vi "Read Sinus penta1.vi"(10 "Parametri inverter 2":T1, 11 "register values":u16[](array[numeric])) -> (2 "output cluster":T1)   [LabVIEW 2019]
uses:
  controls/Parametri inverter letti.ctl
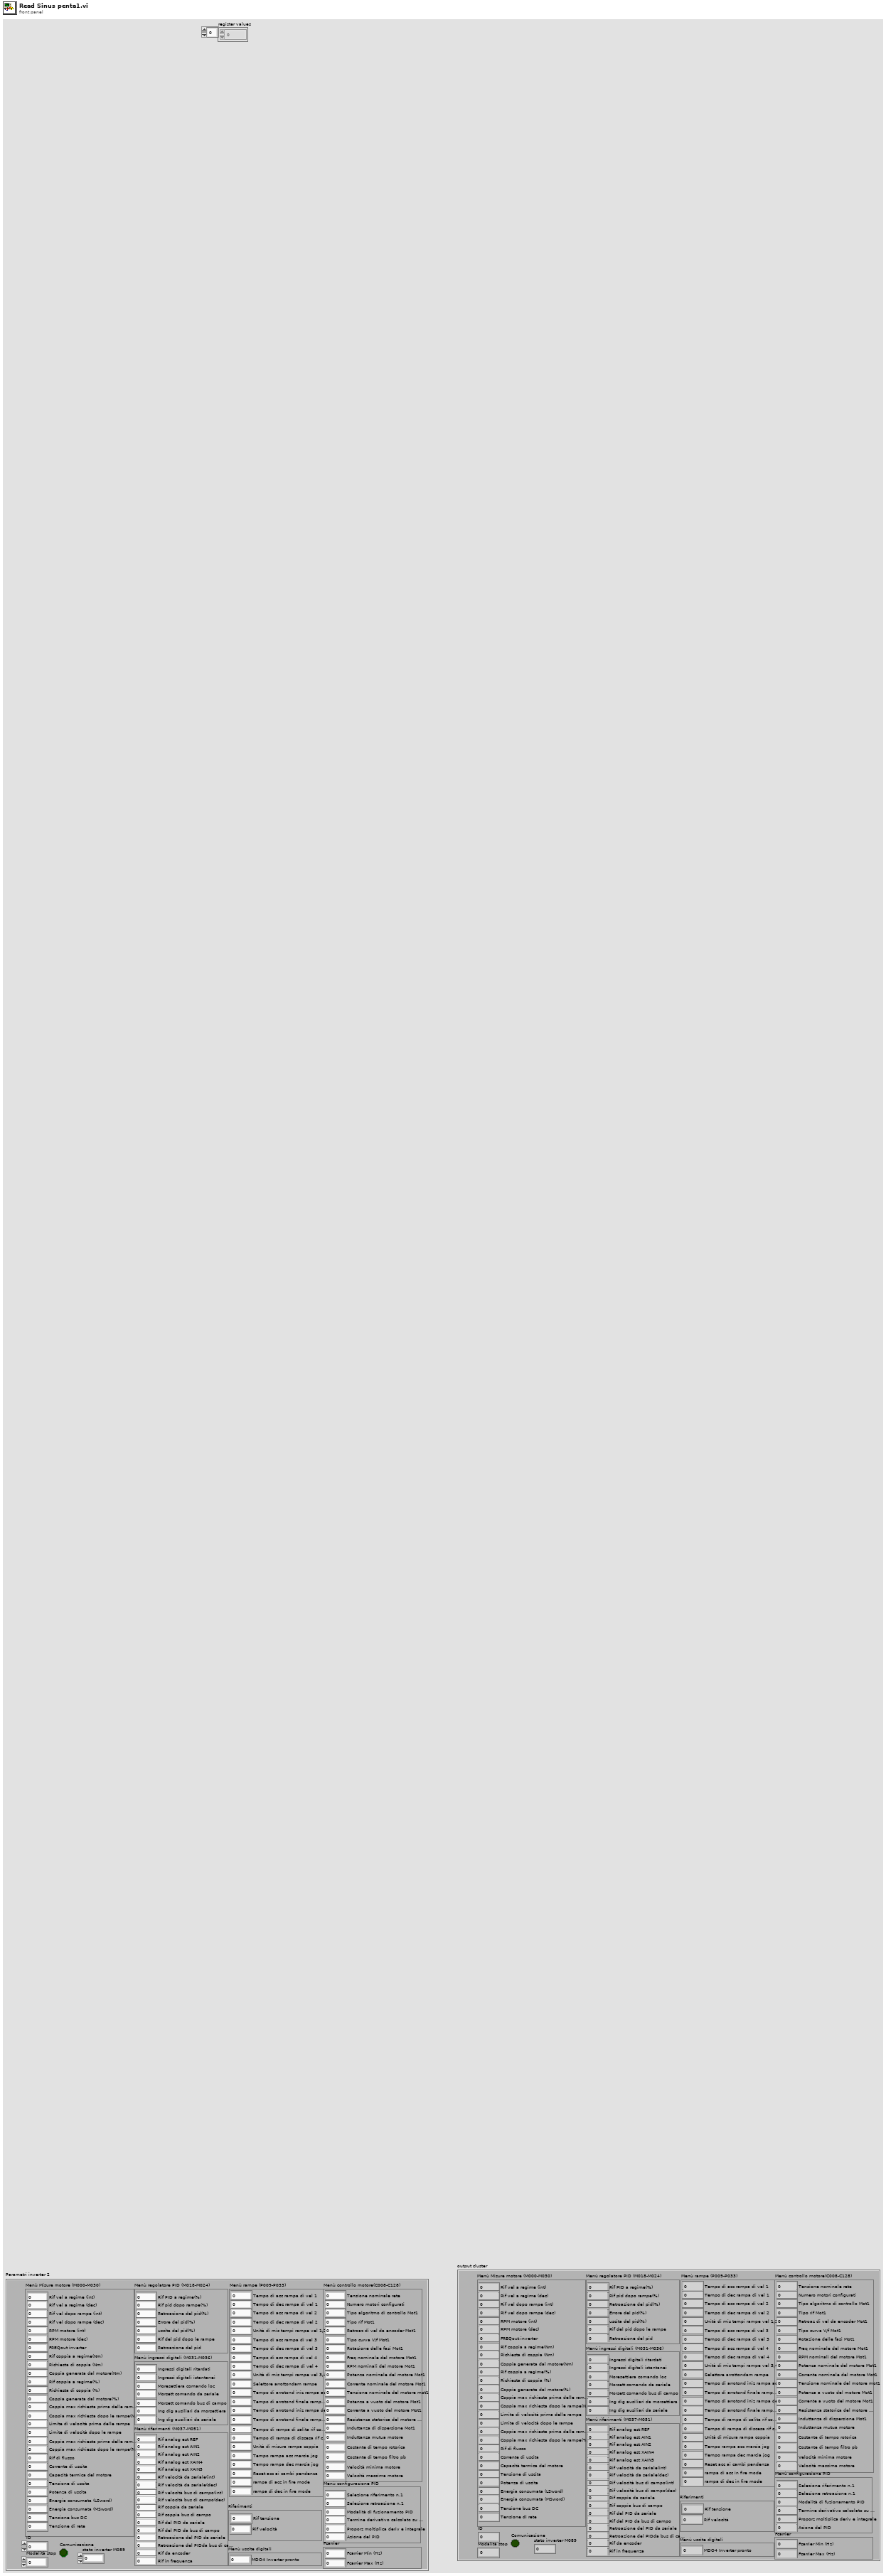
[diagram p1: front panel]
types:
  T1 = typedef "Parametri inverter letti.ctl" = cluster{"Menù Misure motore (M000-M030)":cluster{"Rif vel a regime (int)":u16, "Rif vel a regime (dec)":u16, "Rif vel dopo rampe (int)":u16, "Rif vel dopo rampe (dec)":u16, "RPM motore (int)":u16, "RPM motore (dec)":u16, "FREQout inverter":u16, "Rif coppia a regime(Nm)":u16, "Richiesta di coppia (Nm)":u16, "Coppia generata dal motore(Nm)":u16, "Rif coppia a regime(%)":u16, "Richiesta di coppia (%)":u16, "Coppia generata dal motore(%)":u16, "Coppia max richiesta prima delle rampe(Nm)":u16, "Coppia max richiesta dopo le rampe(Nm)":u16, "Limite di velocità prima delle rampe":u16, "Limite di velocità dopo le rampe":u16, "Coppia max richiesta prima delle rampe(%)":u16, "Coppia max richiesta dopo le rampe(%)":u16, "Rif di flusso":u16, "Corrente di uscita":u16, "Capacità termica del motore":u16, "Tensione di uscita":u16, "Potenza di uscita":u16, "Energia consumata (LSword)":u16, "Energia consumata (MSword)":u16, "Tensione bus DC":u16, "Tensione di rete":u16}, "Menù regolatore PID (M018-M024)":cluster{"Rif PID a regime(%)":u16, "Rif pid dopo rampe(%)":u16, "Retroazione del pid(%)":u16, "Errore del pid(%)":u16, "uscita del pid(%)":u16, "Rif del pid dopo le rampe":u16, "Retroazione del pid":u16}, "Menù ingressi digitali (M031-M036)":cluster{"Ingressi digitali ritardati":u16, "Ingressi digitali istantanei":u16, "Moresettiera comando loc":u16, "Morsett comando da seriale":u16, "Morsett comando bus di campo":u16, "Ing dig ausiliari da morsettiera":u16, "Ing dig ausiliari da seriale":u16}, "Menù riferimenti (M037-M051)":cluster{"Rif analog est REF":u16, "Rif analog est AIN1":u16, "Rif analog est AIN2":u16, "Rif analog est XAIN4":u16, "Rif analog est XAIN5":u16, "Rif velocità da seriale(int)":u16, "Rif velocità bus di campo(int)":u16, "Rif coppia da seriale":u16, "Rif coppia bus di campo":u16, "Rif del PID da seriale":u16, "Rif del PID da bus di campo":u16, "Retroazione del PID da seriale":u16, "Retroazione del PIDda bus di campo":u16, "Rif da encoder":u16, "Rif in frequenza":u16, "Rif velocità da seriale(dec)":u16, "Rif velocità bus di campo(dec)":u16}, "Menù rampe (P009-P033)":cluster{"Tempo di dec rampa di vel 1":u16, "Tempo di acc rampa di vel 2":u16, "Tempo di dec rampa di vel 2":u16, "Tempo di acc rampa di vel 1":u16, "Unità di mis tempi rampe vel 1/2":u16, "Tempo di acc rampa di vel 3":u16, "Tempo di dec rampa di vel 3":u16, "Tempo di acc rampa di vel 4":u16, "Tempo di dec rampa di vel 4":u16, "Unità di mis tempi rampe vel 3/4":u16, "Selettore arrottondam rampe":u16, "Tempo di arrotond iniz rampa acc":u16, "Tempo di arrotond finale rampa acc":u16, "Tempo di arrotond iniz rampa dec":u16, "Tempo di rampa di salita rif coppia":u16, "Tempo di rampa di discesa rif coppia":u16, "Unità di misura rampa coppia":u16, "Tempo rampa acc marcia jog":u16, "Tempo rampa dec marcia jog":u16, "Reset acc ai cambi pendenza":u16, "rampa di acc in fire mode":u16, "rampa di dec in fire mode":u16, "Tempo di arrotond finale rampa dec":u16}, "Menù controllo motore(C008-C128)":cluster{"Numero motori configurati":u16, "Tipo algoritmo di controllo Mot1":u16, "Tipo rif Mot1":u16, "Tensione nominale rete":u16, "Retroaz di vel da encoder Mot1":u16, "Tipo curva V/f Mot1":u16, "Rotazione delle fasi Mot1":u16, "Freq nominale del motore Mot1":u16, "RPM nominali del motore Mot1":u16, "Potenza nominale del motore Mot1":u16, "Corrente nominale del motore Mot1":u16, "Tensione nominale del motore mot1":u16, "Potenza a vuoto del motore Mot1":u16, "Corrente a vuoto del motore Mot1":u16, "Resistenza statorica del motore Mot1":u16, "Induttanza di dispersione Mot1":u16, "Induttanza mutua motore":u16, "Costante di tempo rotorica":u16, "Costante di tempo filtro pb":u16, "Velocità minima motore":u16, "Velocità massima motore":u16}, "Menù configurazione PID":cluster{"Selezione riferimento n.1":u16, "Selezione retroazione n.1":u16, "Modalità di fuzionamento PID":u16, "Termine derivativo calcolato su err o mis":u16, "Proporz moltiplica deriv e integrale":u16, "Azione del PID":u16}, "ID":dbl, "Menù uscite digitali":cluster{"MDO4 Inverter pronto":u16}, "Fcarrier":cluster{"Fcarrier Min (Hz)":u16, "Fcarrier Max (Hz)":u16}, "stato inverter M089":dbl, "Riferimenti":cluster{"Rif tensione":u16, "Rif velocità":u16}, "Comunicazione":bool, "Modalità stop":dbl}
  T2 = cluster{"Rif PID a regime(%)":u16, "Rif pid dopo rampe(%)":u16, "Retroazione del pid(%)":u16, "Errore del pid(%)":u16, "uscita del pid(%)":u16, "Rif del pid dopo le rampe":u16, "Retroazione del pid":u16}
  T3 = cluster{"Ingressi digitali ritardati":u16, "Ingressi digitali istantanei":u16, "Moresettiera comando loc":u16, "Morsett comando da seriale":u16, "Morsett comando bus di campo":u16, "Ing dig ausiliari da morsettiera":u16, "Ing dig ausiliari da seriale":u16}
  T4 = cluster{"Rif vel a regime (int)":u16, "Rif vel a regime (dec)":u16, "Rif vel dopo rampe (int)":u16, "Rif vel dopo rampe (dec)":u16, "RPM motore (int)":u16, "RPM motore (dec)":u16, "FREQout inverter":u16, "Rif coppia a regime(Nm)":u16, "Richiesta di coppia (Nm)":u16, "Coppia generata dal motore(Nm)":u16, "Rif coppia a regime(%)":u16, "Richiesta di coppia (%)":u16, "Coppia generata dal motore(%)":u16, "Coppia max richiesta prima delle rampe(Nm)":u16, "Coppia max richiesta dopo le rampe(Nm)":u16, "Limite di velocità prima delle rampe":u16, "Limite di velocità dopo le rampe":u16, "Coppia max richiesta prima delle rampe(%)":u16, "Coppia max richiesta dopo le rampe(%)":u16, "Rif di flusso":u16, "Corrente di uscita":u16, "Capacità termica del motore":u16, "Tensione di uscita":u16, "Potenza di uscita":u16, "Energia consumata (LSword)":u16, "Energia consumata (MSword)":u16, "Tensione bus DC":u16, "Tensione di rete":u16}
  T5 = cluster{"Rif analog est REF":u16, "Rif analog est AIN1":u16, "Rif analog est AIN2":u16, "Rif analog est XAIN4":u16, "Rif analog est XAIN5":u16, "Rif velocità da seriale(int)":u16, "Rif velocità bus di campo(int)":u16, "Rif coppia da seriale":u16, "Rif coppia bus di campo":u16, "Rif del PID da seriale":u16, "Rif del PID da bus di campo":u16, "Retroazione del PID da seriale":u16, "Retroazione del PIDda bus di campo":u16, "Rif da encoder":u16, "Rif in frequenza":u16, "Rif velocità da seriale(dec)":u16, "Rif velocità bus di campo(dec)":u16}
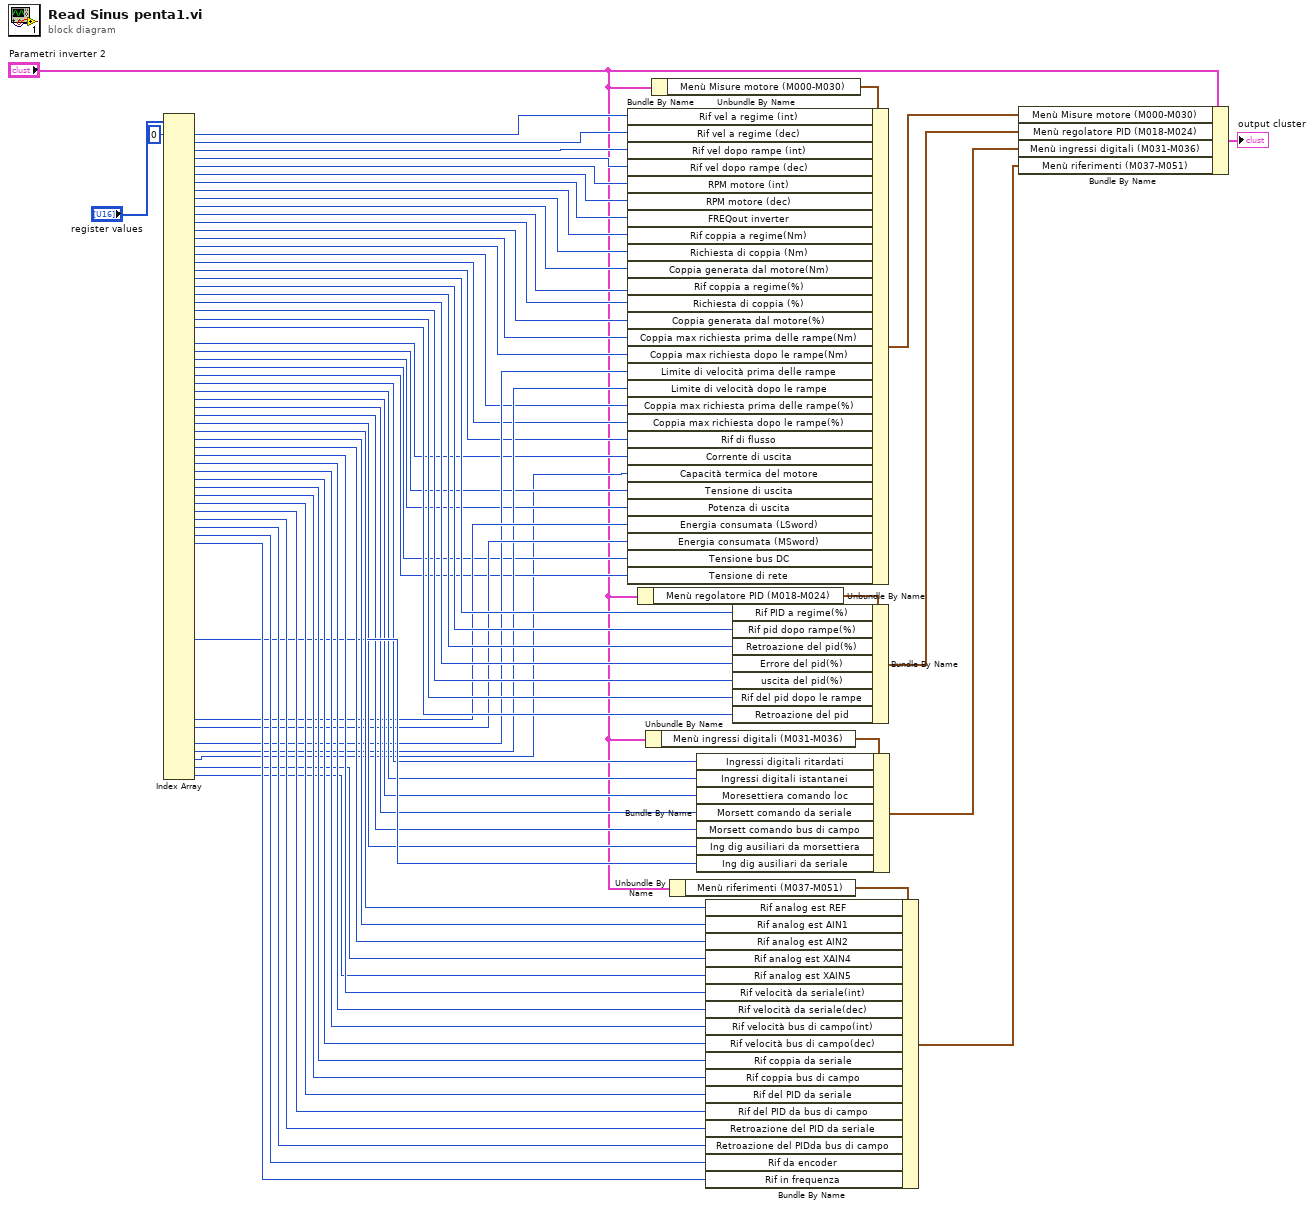
[diagram p0: block diagram]
diagram:
  n1 = Index Array(array="register values", index #1=0 ("index")) -> (element #1=w10:u16, element #2=w11:u16, element #3=w12:u16, element #4=w13:u16, element #5=w15:u16, element #6=w16:u16, element #7=w17:u16, element #8=w18:u16, element #9=w19:u16, element #10=w20:u16, element #11=w21:u16, element #12=w22:u16, element #13=w23:u16, element #14=w24:u16, element #15=w26:u16, element #16=w27:u16, element #17=w28:u16, element #18=w29:u16, element #19=w40:u16, element #20=w41:u16, element #21=w42:u16, element #22=w43:u16, element #23=w44:u16, element #24=w45:u16, element #25=w46:u16, element #27=w30:u16, element #28=w31:u16, element #29=w33:u16, element #30=w32:u16, element #31=w34:u16, element #32=w48:u16, element #33=w49:u16, element #34=w50:u16, element #35=w51:u16, element #36=w52:u16, element #37=w53:u16, element #38=w56:u16, element #39=w57:u16, element #40=w58:u16, element #41=w60:u16, element #42=w61:u16, element #43=w62:u16, element #44=w63:u16, element #45=w64:u16, element #46=w65:u16, element #47=w66:u16, element #48=w67:u16, element #49=w68:u16, element #50=w69:u16, element #51=w70:u16, element #52=w71:u16, element #64=w54:u16, element #74=w38:u16, element #75=w37:u16, element #77=w35:u16, element #78=w36:u16, element #79=w4:u16, element #80=w59:u16, element #81=w3:u16)  [unwired: 80 in, 22 out]
  n2 = Unbundle By Name("Parametri inverter 2") -> ("Menù regolatore PID (M018-M024)"=w39:T2)
  n3 = Unbundle By Name("Parametri inverter 2") -> ("Menù ingressi digitali (M031-M036)"=w47:T3)
  n4 = Unbundle By Name("Parametri inverter 2") -> ("Menù Misure motore (M000-M030)"=w25:T4)
  n5 = Bundle By Name(cluster=w25, "Rif vel a regime (int)"=w10, "Rif vel a regime (dec)"=w11, "Rif vel dopo rampe (int)"=w12, "Rif vel dopo rampe (dec)"=w13, "RPM motore (int)"=w15, "RPM motore (dec)"=w16, "FREQout inverter"=w17, "Rif coppia a regime(Nm)"=w18, "Richiesta di coppia (Nm)"=w19, "Coppia generata dal motore(Nm)"=w20, "Rif coppia a regime(%)"=w21, "Richiesta di coppia (%)"=w22, "Coppia generata dal motore(%)"=w23, "Coppia max richiesta prima delle rampe(Nm)"=w24, "Coppia max richiesta dopo le rampe(Nm)"=w26, "Limite di velocità prima delle rampe"=w35, "Limite di velocità dopo le rampe"=w36, "Coppia max richiesta prima delle rampe(%)"=w27, "Coppia max richiesta dopo le rampe(%)"=w28, "Rif di flusso"=w29, "Corrente di uscita"=w30, "Capacità termica del motore"=w4, "Tensione di uscita"=w31, "Potenza di uscita"=w33, "Energia consumata (LSword)"=w38, "Energia consumata (MSword)"=w37, "Tensione bus DC"=w32, "Tensione di rete"=w34) -> (w8:T4)
  n6 = Unbundle By Name("Parametri inverter 2") -> ("Menù riferimenti (M037-M051)"=w55:T5)
  n7 = Bundle By Name(cluster=w47, "Ingressi digitali ritardati"=w48, "Ingressi digitali istantanei"=w49, "Moresettiera comando loc"=w50, "Morsett comando da seriale"=w51, "Morsett comando bus di campo"=w52, "Ing dig ausiliari da morsettiera"=w53, "Ing dig ausiliari da seriale"=w54) -> (w6:T3)
  n8 = Bundle By Name(cluster=w55, "Rif analog est REF"=w56, "Rif analog est AIN1"=w57, "Rif analog est AIN2"=w58, "Rif analog est XAIN4"=w59, "Rif analog est XAIN5"=w3, "Rif velocità da seriale(int)"=w60, "Rif velocità da seriale(dec)"=w61, "Rif velocità bus di campo(int)"=w62, "Rif velocità bus di campo(dec)"=w63, "Rif coppia da seriale"=w64, "Rif coppia bus di campo"=w65, "Rif del PID da seriale"=w66, "Rif del PID da bus di campo"=w67, "Retroazione del PID da seriale"=w68, "Retroazione del PIDda bus di campo"=w69, "Rif da encoder"=w70, "Rif in frequenza"=w71) -> (w5:T5)
  n9 = Bundle By Name(cluster=w39, "Rif PID a regime(%)"=w40, "Rif pid dopo rampe(%)"=w41, "Retroazione del pid(%)"=w42, "Errore del pid(%)"=w43, "uscita del pid(%)"=w44, "Rif del pid dopo le rampe"=w45, "Retroazione del pid"=w46) -> (w7:T2)
  n10 = Bundle By Name(cluster="Parametri inverter 2", "Menù Misure motore (M000-M030)"=w8, "Menù regolatore PID (M018-M024)"=w7, "Menù ingressi digitali (M031-M036)"=w6, "Menù riferimenti (M037-M051)"=w5) -> (→"output cluster":T1)
